vi "Test_TextFileSink_CreateandWritetoFile_FileExistsAndValidData.vi"(8 "error in (no error)":errorcluster, 11 "TestCase in":refnum<class "TestTextFileSink.lvclass">) -> (0 "error out":errorcluster, 3 "TestCase out":refnum<class "TestTextFileSink.lvclass">)   [LabVIEW 2017, in "TestTextFileSink.lvclass"]
uses:
  TestTextFileSink.lvclass
  Source/Text File Sink/Configuration.ctl
  Source/Composed Log/LoggerReference/LoggerReference.lvclass/LoggerReference.ctl
  e024c6b3-4803-40b0-907f-2d7f922acde5.vi
  Source/Composed Log/LoggerReference/Return Aggregate Queues.vi
  Source/Composed Log/LoggerReference/Add Aggregate Log.vi
  e024c6b3-4803-40b0-907f-2d7f922acde5.vi/4c0b7c79-22e1-4909-99f8-25ae8e89444c.vi
  Source/Composed Log/LoggerReference/Log.vi
  Source/Composed Log/LoggerReference/Send Add Sink.vi
  Source/Composed Log/LoggerReference/Remove Stale Logs.vi
  Source/Text File Sink/Text File Sink.lvclass
  C:/CS/Internal/LabVIEW/Logger/Source/Composed Log/Log Sink/Log Sink.lvclass
  Source/Composed Log/Application Logger/Launch Worker Loop.vi
  Source/Composed Log/LoggerReference/Initialize Logger Instance.vi
  Source/Composed Log/LoggerReference/LoggerReference.lvclass
  Source/Composed Log/IErrorFormat/IErrorFormat.lvclass
  Source/Composed Log/Log Sink/Log Sink.lvclass
  <vilib>/addons/_JKI Toolkits/VI Tester/TestCase.llb/TestCase.lvclass
  C:/Program Files (x86)/National Instruments/LabVIEW 2017/vi.lib/addons/_JKI Toolkits/VI Tester/TestCase.llb/TestCase.lvclass
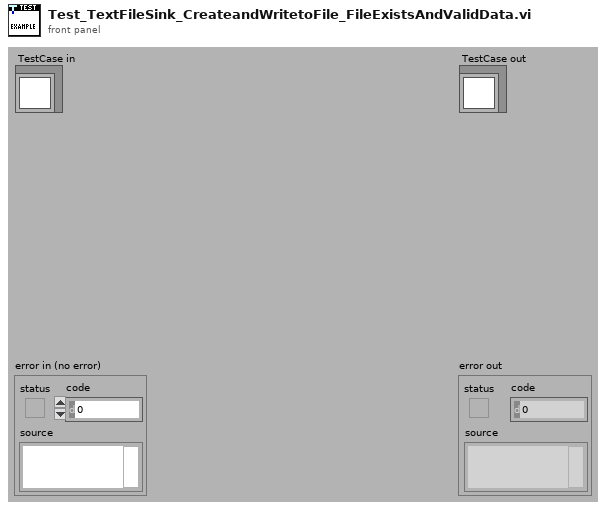
[diagram p1: front panel]
types:
  T1 = typedef "Text File Sink.lvclass/Configuration.ctl" = cluster{"Folder":path, "Name":string, "Extension":string, "Max Size (MB)":i64, "Timestamp Filename":bool}
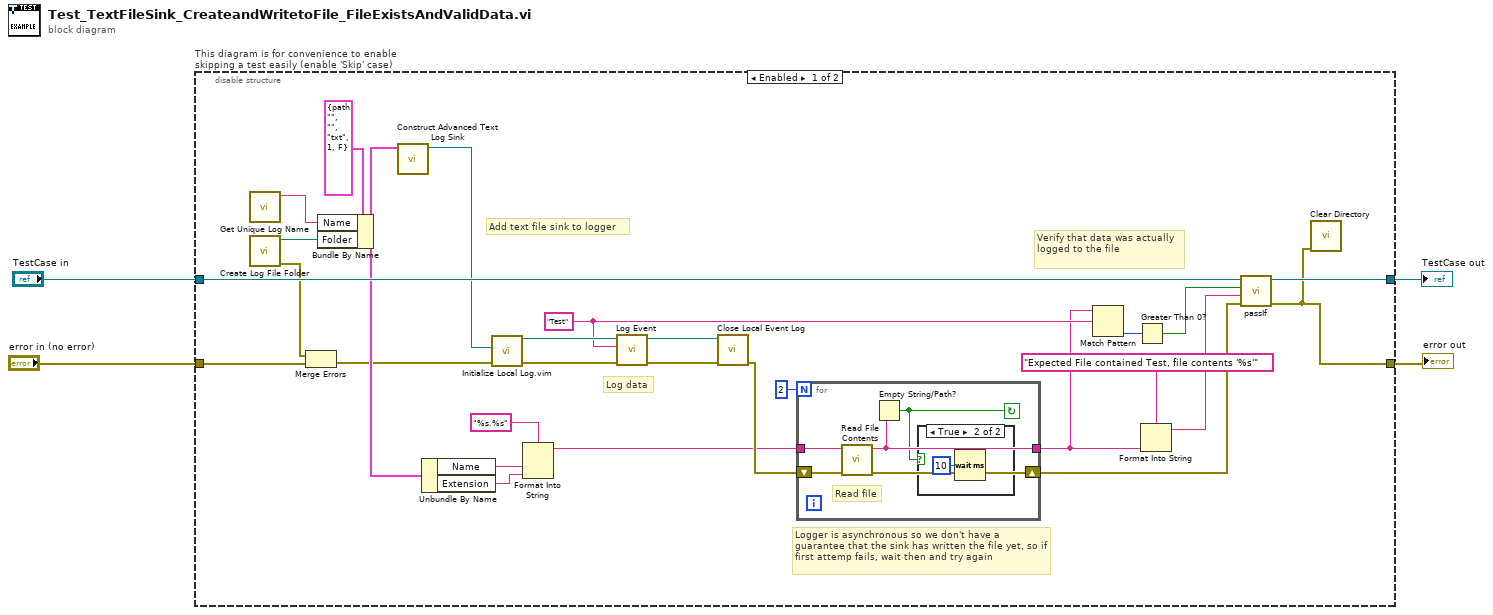
[diagram p0: block diagram]
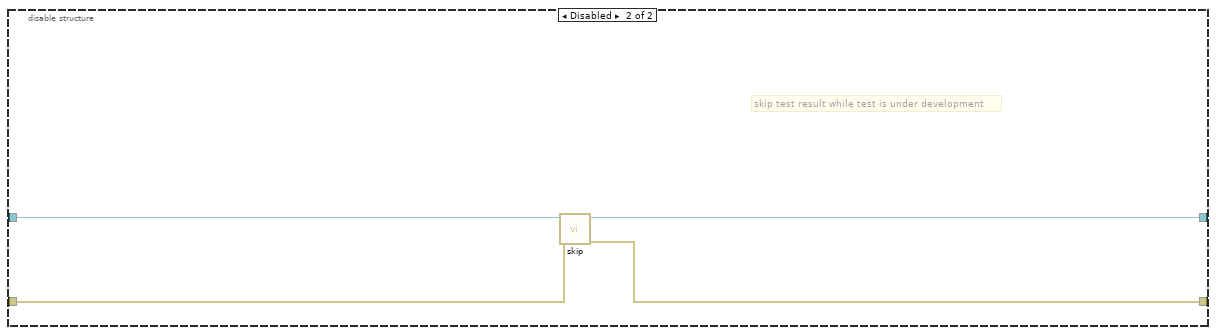
[diagram p3: hidden frame]
diagram:
  n1 = disable-structure "This diagram is for convenience to enable skipping a test easily (enable 'Skip' case)" shown="Enabled" {
    disable-tunnel: "TestCase in" -> [w31 w42]
    disable-tunnel: [w30 w40] -> w1
    disable-tunnel: [w29 w41] -> w3
    disable-tunnel: "error in (no error)" -> [w32 w39]
    frame Enabled {
      w19 = "Test" ("SourceID")
      # "Logger is asynchronous so we don't have a guarantee that the sink has written the file yet, so if first attemp fails, wait then and try again"
      # "Verify that data was actually logged to the file"
      # "Log data"
      # "Add text file sink to logger"
      n2 = call "Get Unique Log Name.vi"() -> ("Log File Name"=w10:string)  [unwired: 11 in]
      n3 = call "Create Log File Folder.vi"() -> ("error out"=w11:errorcluster, "Folder Path"=w27:path)  [unwired: 10 in]
      n4 = Merge Errors(w11, w32) -> (w12:errorcluster)
      n5 = Bundle By Name(cluster=T1 {"Folder"=path "", "Name"="", "Extension"="txt", "Max Size (MB)"=1, "Timestamp Filename"=FALSE} ("Text File Configuration"), "Name"=w10, "Folder"=w27) -> (w17:T1)
      n6 = call "Construct Advanced Text Log Sink.vi"("Text File Configuration"=w17) -> ("Text File Sink out"=w26:refnum<class "Text File Sink.lvclass">)  [unwired: 10 in]
      n7 = Unbundle By Name(w17) -> ("Name"=w15:string, "Extension"=w14:string)
      n8 = call "Initialize Local Log.vim"("error in (no error)"=w12, "Startup Sink(s)"=w26) -> ("error out"=w25:errorcluster, "Log Instance Reference"=w24:refnum<class "LoggerReference.lvclass">)  [unwired: 7 in, 1 out]
      n9 = Format Into String(format string="%s.%s", w15, w14) -> (resulting string=w13:string)  [unwired: 2 in, 1 out]
      n10 = call "Log Event.vi"("error in (no error)"=w25, "SourceID"=w19, "Log Instance"=w24) -> ("error out"=w23:errorcluster, "Log Instance Out"=w22:refnum<class "LoggerReference.lvclass">)  [unwired: 7 in]
      n11 = call "Close Local Event Log.vi"("error in (no error)"=w23, "Log Instance"=w22) -> ("error out"=w21:errorcluster)  [unwired: 9 in]
      n12 = for {
        N: 2 -> [_]
        shift-right: [w36] -> w20
        shift-left: w21 -> [w37]
        tunnel: w13 -> [w35]
        tunnel: [w34] -> w8
        stop <- w33 continue-if-true
        # "Read file"
        n13 = call "Read File Contents.vi"("error in (no error)"=w37, "File Name"=w35) -> ("error out"=w36:errorcluster, "File Text"=w34:string)  [unwired: 8 in]
        n14 = Empty String/Path?(string/path=w34) -> (empty?=w33:bool)
        n15 = case shown="True" w33 {
          frame False {
          }
          frame True {
            n16 = Wait (ms)(milliseconds to wait=u32 10) -> ()  [unwired: 1 out]
          }
        }
      }
      n17 = Match Pattern(string=w8, regular expression=w19) -> (offset past match=w18:i32)  [unwired: 1 in, 3 out]
      n18 = Greater Than 0?(x=w18) -> (x > 0?=w6:bool)
      n19 = Format Into String(format string="Expected File contained Test, file contents '%s'", w8) -> (resulting string=w7:string)  [unwired: 2 in, 1 out]
      n20 = call-dynamic "passIf.vi"("error in (no error)"=w20, "message (\"\")"=w7, "pass"=w6, "TestCase in"=w31) -> ("error out"=w29:errorcluster, "TestCase out"=w30:refnum<class "TestTextFileSink.lvclass">)  [unwired: 6 in]
      n21 = call "Clear Directory.vi"("error in"=w29) -> ()  [unwired: 10 in, 1 out]
    }
    frame Disabled {
      # "skip test result while test is under development"
      n22 = call <vilib>:"skip.vi"("error in (no error)"=w39, "TestCase in"=w42) -> ("error out"=w41:errorcluster, "TestCase out"=w40:refnum<class "TestTextFileSink.lvclass">)  [unwired: 8 in]
    }
  }
  "error out" <- w3
  "TestCase out" <- w1
